vi "DecodeStatus SubVI.vi"(2 "S2":u8, 3 "S1":u8) -> (0 "S2 String":string, 1 "S1 String":string)   [LabVIEW 2019]
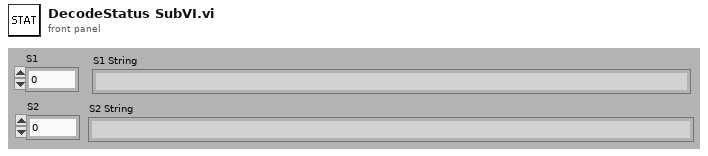
[diagram p1: front panel]
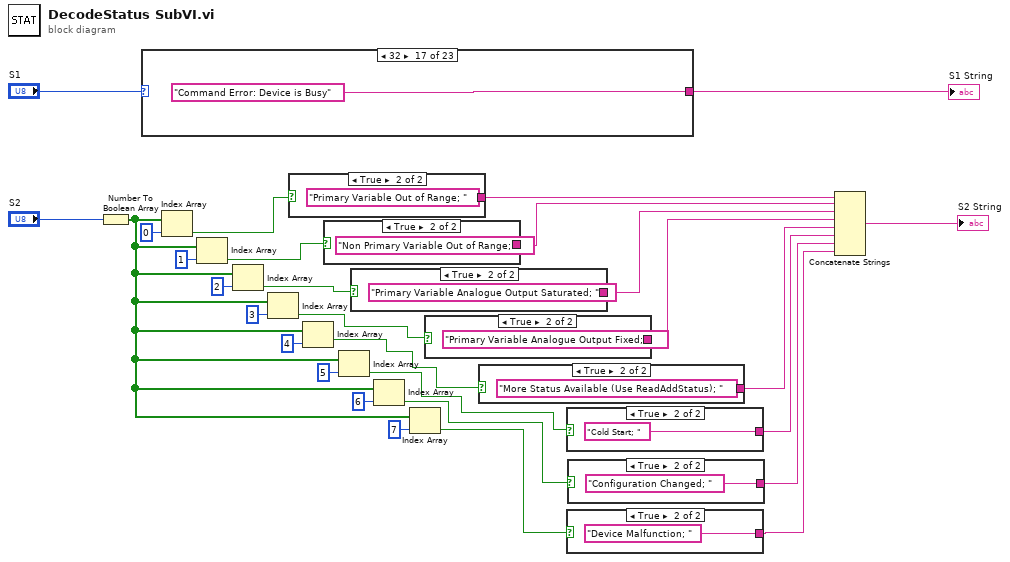
[diagram p0: block diagram]
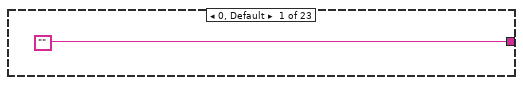
[diagram p2: hidden frame]
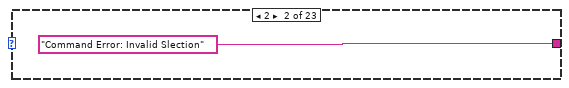
[diagram p3: hidden frame]
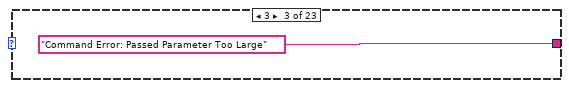
[diagram p4: hidden frame]
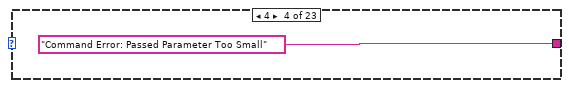
[diagram p5: hidden frame]
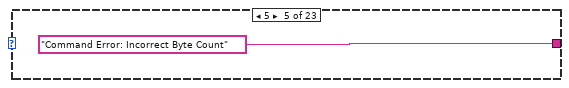
[diagram p6: hidden frame]
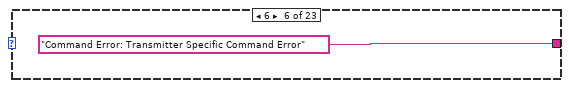
[diagram p7: hidden frame]
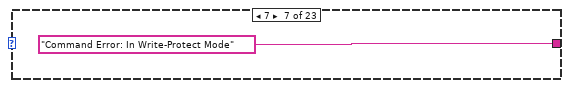
[diagram p8: hidden frame]
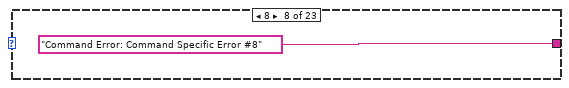
[diagram p9: hidden frame]
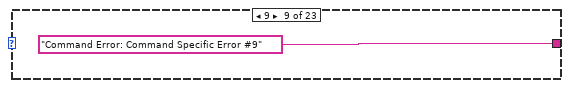
[diagram p10: hidden frame]
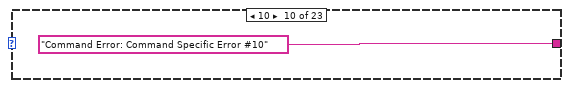
[diagram p11: hidden frame]
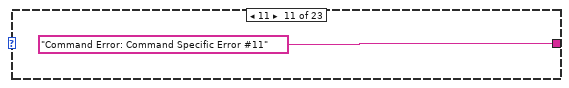
[diagram p12: hidden frame]
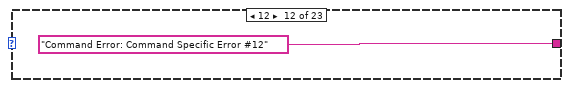
[diagram p13: hidden frame]
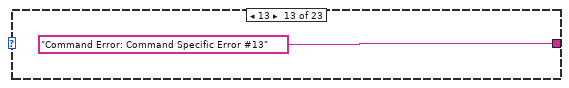
[diagram p14: hidden frame]
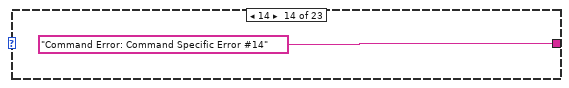
[diagram p15: hidden frame]
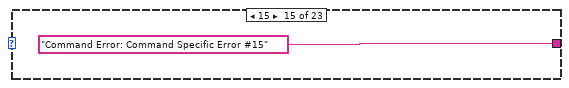
[diagram p16: hidden frame]
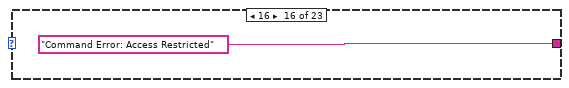
[diagram p17: hidden frame]
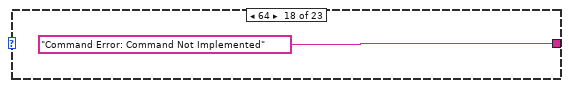
[diagram p18: hidden frame]
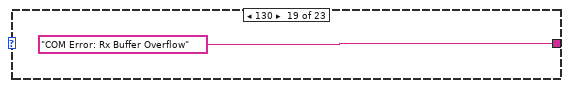
[diagram p19: hidden frame]
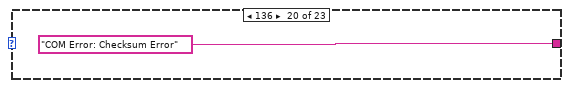
[diagram p20: hidden frame]
diagram:
  n1 = Number To Boolean Array(number="S2") -> (Boolean array=w11:bool[])
  n2 = case shown="32" "S1" {
    tunnel: ["" "Command Error: Invalid Slection" "Command Error: Passed Parameter Too Large" "Command Error: Passed Parameter Too Small" "Command Error: Incorrect Byte Count" "Command Error: Transmitter Specific Command Error" "Command Error: In Write-Protect Mode" "Command Error: Command Specific Error #8" "Command Error: Command Specific Error #9" "Command Error: Command Specific Error #10" "Command Error: Command Specific Error #11" "Command Error: Command Specific Error #12" "Command Error: Command Specific Error #13" "Command Error: Command Specific Error #14" "Command Error: Command Specific Error #15" "Command Error: Access Restricted" "Command Error: Device is Busy" "Command Error: Command Not Implemented" "COM Error: Rx Buffer Overflow" "COM Error: Checksum Error" "COM Error: Framing Error" "COM Error: Overrun Error" "COM Error: Parity Error"] -> w29
    frame 0, Default {
    }
    frame 2 {
    }
    frame 3 {
    }
    frame 4 {
    }
    frame 5 {
    }
    frame 6 {
    }
    frame 7 {
    }
    frame 8 {
    }
    frame 9 {
    }
    frame 10 {
    }
    frame 11 {
    }
    frame 12 {
    }
    frame 13 {
    }
    frame 14 {
    }
    frame 15 {
    }
    frame 16 {
    }
    frame 32 {
    }
    frame 64 {
    }
    frame 130 {
    }
    frame 136 {
    }
    frame 144 {
    }
    frame 160 {
    }
    frame 192 {
    }
  }
  "S1 String" <- w29
  n3 = Index Array(array=w11, index=0) -> (element=w12:bool)
  n4 = Index Array(array=w11, index=1) -> (element=w13:bool)
  n5 = Index Array(array=w11, index=2) -> (element=w14:bool)
  n6 = Index Array(array=w11, index=3) -> (element=w15:bool)
  n7 = case shown="True" w12 {
    tunnel: ["" "Primary Variable Out of Range; "] -> w20
    frame False {
    }
    frame True {
    }
  }
  n8 = Index Array(array=w11, index=4) -> (element=w16:bool)
  n9 = case shown="True" w13 {
    tunnel: ["" "Non Primary Variable Out of Range; "] -> w21
    frame False {
    }
    frame True {
    }
  }
  n10 = Index Array(array=w11, index=5) -> (element=w17:bool)
  n11 = case shown="True" w14 {
    tunnel: ["" "Primary Variable Analogue Output Saturated; "] -> w22
    frame False {
    }
    frame True {
    }
  }
  n12 = Index Array(array=w11, index=6) -> (element=w18:bool)
  n13 = Index Array(array=w11, index=7) -> (element=w19:bool)
  n14 = case shown="True" w15 {
    tunnel: ["" "Primary Variable Analogue Output Fixed; "] -> w23
    frame False {
    }
    frame True {
    }
  }
  n15 = case shown="True" w16 {
    tunnel: ["" "More Status Available (Use ReadAddStatus); "] -> w24
    frame False {
    }
    frame True {
    }
  }
  n16 = case shown="True" w17 {
    tunnel: ["" "Cold Start; "] -> w25
    frame False {
    }
    frame True {
    }
  }
  n17 = case shown="True" w19 {
    tunnel: ["" "Device Malfunction; "] -> w27
    frame False {
    }
    frame True {
    }
  }
  n18 = case shown="True" w18 {
    tunnel: ["" "Configuration Changed; "] -> w26
    frame False {
    }
    frame True {
    }
  }
  n19 = Concatenate Strings(w20, w21, w22, w23, w24, w25, w26, w27) -> (→"S2 String":string)
